vi "FB Global Strings.vi"() -> ()   [LabVIEW 2020]
panel:
  in  "ConfigurationPage::Typedef":string="Type definition"
  in  "Errors":cluster{"Error":string, "Details":string}[](array[cluster])=[{"Error"="No Owning Project", "Details"="The function block must be opened in a project."}, {"Error"="Created Without Owning Project", "Details"="A function block can be used only in a standard VI that is part of a LabVIEW project. Delete the function block, and create a new function block in a VI that is part of a LabVIEW project. \n\nA function block cannot be used in a SubSystem VI or Statechart Diagram. To use a function block in one of these environments, add the function block to a standard VI in a LabVIEW project and call that VI from the SubSystem VI or Statechart Diagram."}]
  in  "ConfigurationPage::Refnum not supported":string="Refnum type not supported"
  in  "ConfigurationPage::I/O Named Control":string="I/O Named Control"
  in  "ConfigurationPage::Motion Resource":string="Motion Resource"
  in  "ConfigurationPage::No Owning Project":string="Cannot configure function block properties. To configure function block properties, the function block must be created and opened in a project."
  in  "ConfigurationPage::Tag":string="Tag"
  in  "ConfigurationPage::Refnum":string="Refnum"
  in  "ConfigurationPage::Array":string="Array"
  in  "ConfigurationPage::Cluster":string="Cluster"
  in  "Popup menu::Polymorphic instances":string="Polymorphic instances"
  in  "ConfigurationPage::Select a VI":string="Select a VI"
  in  "Wizard::error out.code":string="error out.code"
  in  "Wizard::error in.code":string="error in.code"
  in  "Wizard::error out.status":string="error out.status"
  in  "Wizard::error in.status":string="error in.status"
  in  "Wizard::Instance Name":string="My Function Block"
  in  "InstanceNameChange::Message":string="'%s' is in use by another Function Block. Would you like to use '%s' instead?"
  in  "InstanceNameChange::No":string="No, cancel name change"
  in  "InstanceNameChange::Yes":string="Yes, use suggested name"
  in  "ConfigurationPage::Boolean::False":string="FALSE"
  in  "ConfigurationPage::Boolean::True":string="TRUE"
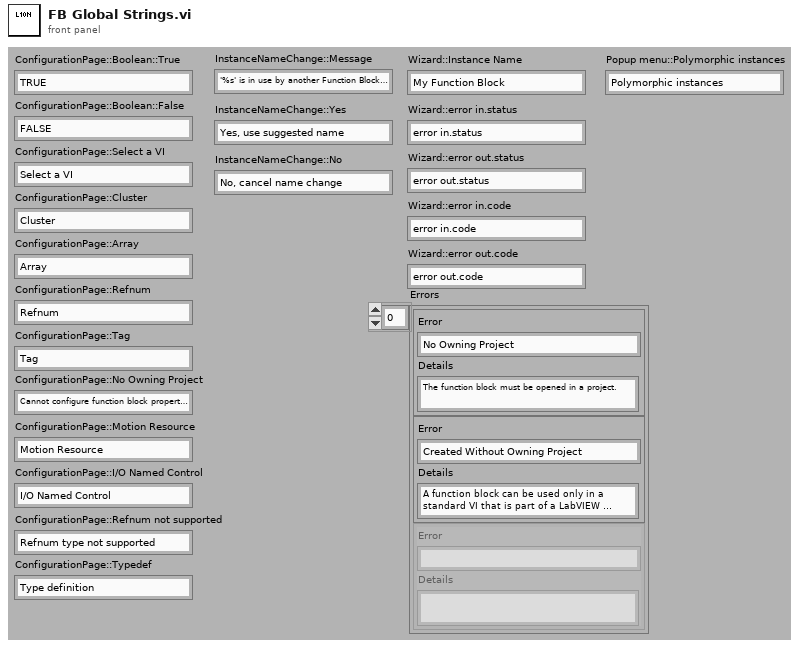
[diagram p1: front panel]
diagram:
